vi "K6221-FreqSweep.vi"   [LabVIEW 2016]
uses:
  Global/Global Variables/global.vi
  Instrument_Setup.vi
  Global/Global Variables/Data_Display_global.vi
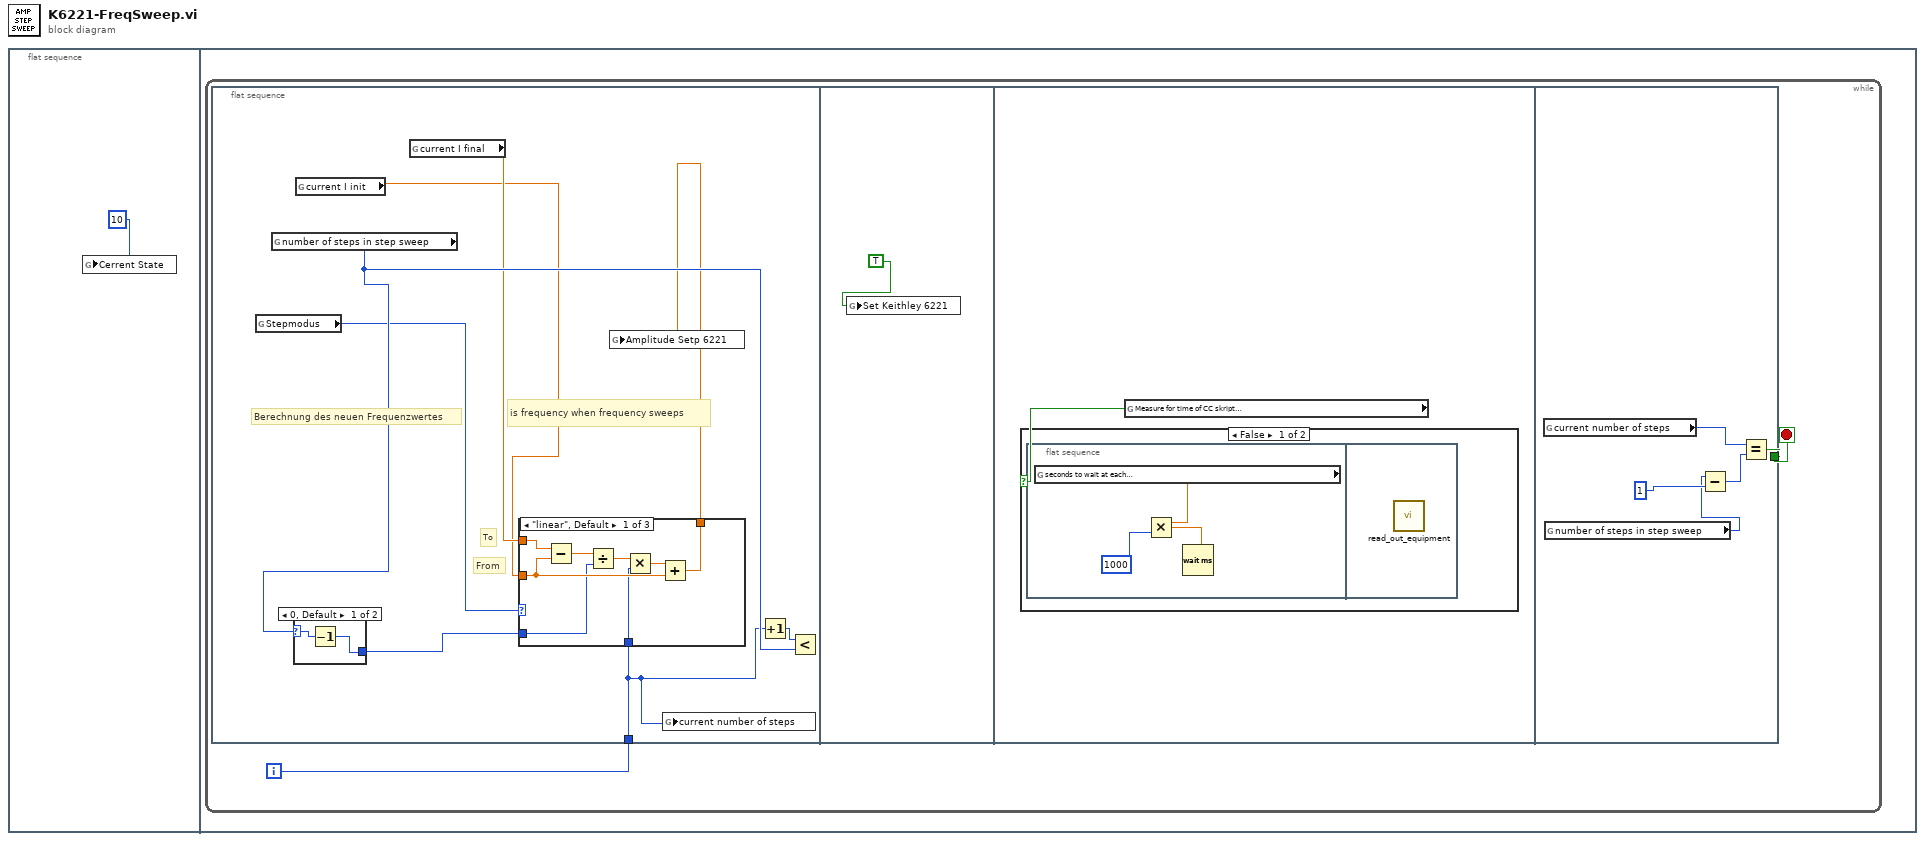
[diagram p0: block diagram]
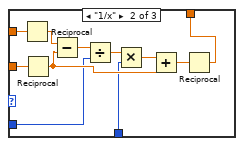
[diagram p3: hidden frame]
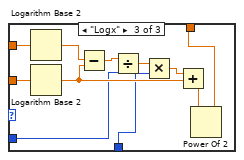
[diagram p4: hidden frame]
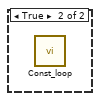
[diagram p5: hidden frame]
diagram:
  n1 = flat-sequence {
    frame #0 {
      n2 = global write "global.vi" "Cerrent State"(10) -> ()
    }
    frame #1 {
      n3 = while {
        i -> [w2]
        stop <- w3 stop-if-true
        n4 = flat-sequence {
          tunnel: w2 -> [w4]
          tunnel: [w53] -> w3
          frame #0 {
            # "From"
            # "To"
            # "is frequency when frequency sweeps"
            # "Berechnung des neuen Frequenzwertes"
            n5 = global read "Instrument_Setup.vi" "Stepmodus"() -> (w8:enum16{"linear", "1/x", "Logx"})
            n6 = global read "global.vi" "number of steps in step sweep"() -> (w9:i32)
            n7 = case shown="0, Default" w9 {
              selector: w9 -> [w13 w14]
              tunnel: [w12 w14] -> w10
              frame 0, Default {
                n8 = Decrement(x=w13) -> (x-1=w12:i32)
              }
              frame 1 {
              }
            }
            n9 = global read "global.vi" "current I init"() -> (w5:dbl)
            n10 = global read "global.vi" "current I final"() -> (w7:dbl)
            n11 = case shown="\"linear\", Default" w8 {
              tunnel: w7 -> [w22 w32 w44]
              tunnel: w5 -> [w19 w33 w43]
              tunnel: [w17 w27 w36] -> w6
              tunnel: w10 -> [w16 w24 w35]
              tunnel: w4 -> [w15 w23 w34]
              frame "linear", Default {
                n12 = Subtract(x=w22, y=w19) -> (x-y=w21:dbl)
                n13 = Divide(x=w21, y=w16) -> (x/y=w20:dbl)
                n14 = Multiply(x=w20, y=w15) -> (x*y=w18:dbl)
                n15 = Add(x=w18, y=w19) -> (x+y=w17:dbl)
              }
              frame "1/x" {
                n16 = Reciprocal(x=w32) -> (1/x=w26:dbl)
                n17 = Reciprocal(x=w33) -> (1/x=w25:dbl)
                n18 = Subtract(x=w26, y=w25) -> (x-y=w31:dbl)
                n19 = Divide(x=w31, y=w24) -> (x/y=w30:dbl)
                n20 = Multiply(x=w30, y=w23) -> (x*y=w29:dbl)
                n21 = Add(x=w29, y=w25) -> (x+y=w28:dbl)
                n22 = Reciprocal(x=w28) -> (1/x=w27:dbl)
              }
              frame "Logx" {
                n23 = Logarithm Base 2(1:w44) -> (0:w42:dbl)
                n24 = Logarithm Base 2(1:w43) -> (0:w38:dbl)
                n25 = Subtract(x=w42, y=w38) -> (x-y=w41:dbl)
                n26 = Divide(x=w41, y=w35) -> (x/y=w40:dbl)
                n27 = Multiply(x=w40, y=w34) -> (x*y=w39:dbl)
                n28 = Add(x=w39, y=w38) -> (x+y=w37:dbl)
                n29 = Power Of 2(x=w37) -> (2^x=w36:dbl)
              }
            }
            n30 = global write "Data_Display_global.vi" "Amplitude Setp 6221"(w6) -> ()
            n31 = global write "Data_Display_global.vi" "current number of steps"(w4) -> ()
            n32 = Increment(x=w4) -> (x+1=w11:i32)
            n33 = Less?(x=w11, y=w9) -> ()  [unwired: 1 out]
          }
          frame #1 {
            n34 = global write "Data_Display_global.vi" "Set Keithley 6221"(TRUE) -> ()
          }
          frame #2 {
            n35 = global read "Instrument_Setup.vi" "Measure for time of CC skript\nat each field step point"() -> (w46:bool)
            n36 = case shown="False" w46 {
              frame False {
                n37 = flat-sequence {
                  frame #0 {
                    n38 = global read "Instrument_Setup.vi" "seconds to wait at each\ncurrent step in a I-step sweep"() -> (w49:dbl)
                    n39 = Multiply(x=w49, y=u32 1000 ("milliseconds to wait")) -> (x*y=w47:dbl)
                    n40 = Wait (ms)(milliseconds to wait=w47) -> ()  [unwired: 1 out]
                  }
                  frame #1 {
                    n41 = call "read_out_equipment.vi"() -> ()  [unwired: 1 in]
                  }
                }
              }
              frame True {
                n42 = call "Const_loop.vi"() -> ()  [unwired: 4 in]
              }
            }
          }
          frame #3 {
            n43 = global read "Data_Display_global.vi" "current number of steps"() -> (w54:i32)
            n44 = global read "global.vi" "number of steps in step sweep"() -> (w51:i32)
            n45 = Subtract(x=w51, y=1) -> (x-y=w50:i32)
            n46 = Equal?(x=w54, y=w50) -> (x = y?=w53:bool)
          }
        }
      }
    }
  }
